vi "DAQ - Append NEW Data.vi"(0 "reference in":refnum<class "GSwFormDSP.lvclass">, 5 "error in (no error)":errorcluster, 7 "New Data":waveform(dbl)[](array[waveform])) -> (11 "Last Values":string[](array[string]), 13 "Time Offset":dbl, 14 "reference out":refnum<class "GSwFormDSP.lvclass">, 16 "Save to File":bool, 19 "error out":errorcluster)   [LabVIEW 2020, in "GSwFormDSP.lvclass"]
uses:
  GSwFormDSP.lvclass
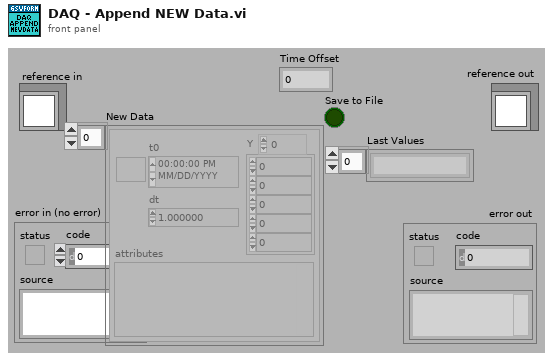
[diagram p1: front panel]
types:
  T1 = typedef "GSwFormDSP.lvclass/ObjectAttributes.ctl" = cluster{"Wform Ref":refnum<data-value>, "Nb Signals":i32, "Spectral Function Parameters":T2, "FFT":waveform(cdb)[], "Nb FFT":i32, "Nb Averages":i32[], "Reference Indexes":i32[], "Response Indexes":i32[], "Coherence":waveform(dbl)[], "TDF Parameters":T4, "DAQ":cluster{"Duration (sec)":dbl, "Buffer Size (Samples)":i32, "Offset (Samples)":i32}, "Filter Impulse Response (TDF)":waveform(dbl), "Sound Playback":T5}
  T2 = typedef "GSwFormDSP.lvclass/Spectral Parameters.ctl" = cluster{"Frequency resolution (Hz)":dbl, "Overlap":dbl, "Window":T3}
  T3 = typedef "NI_AALPro.lvlib/windowTd.ctl" = u32
  T4 = typedef "GSwFormDSP.lvclass/TDF Parameters.ctl" = cluster{"Filter":enum32{"Lowpass", "Highpass", "Bandpass", "Bandstop"}, "Type:":enum16{"Butterworth", "Chebyshev", "Inv Chebyshev", "Elliptic", "Bessel"}, "LP cutoff freq":dbl, "HP cutoff freq":dbl, "Order":i32, "passband ripple (dB)":dbl, "stopband attenuation (dB)":dbl, "Phaseless Filter":bool, "Include Fade IN and OUT":bool}
  T5 = typedef "GSwFormDSP.lvclass/Sound Playback.ctl" = cluster{"Timer start (ms)":u32, "task ID":T6, "Cursor Init Location (s)":dbl, "SC Volume":dbl}
  T6 = typedef "Sound Output Task ID.ctl" = u32
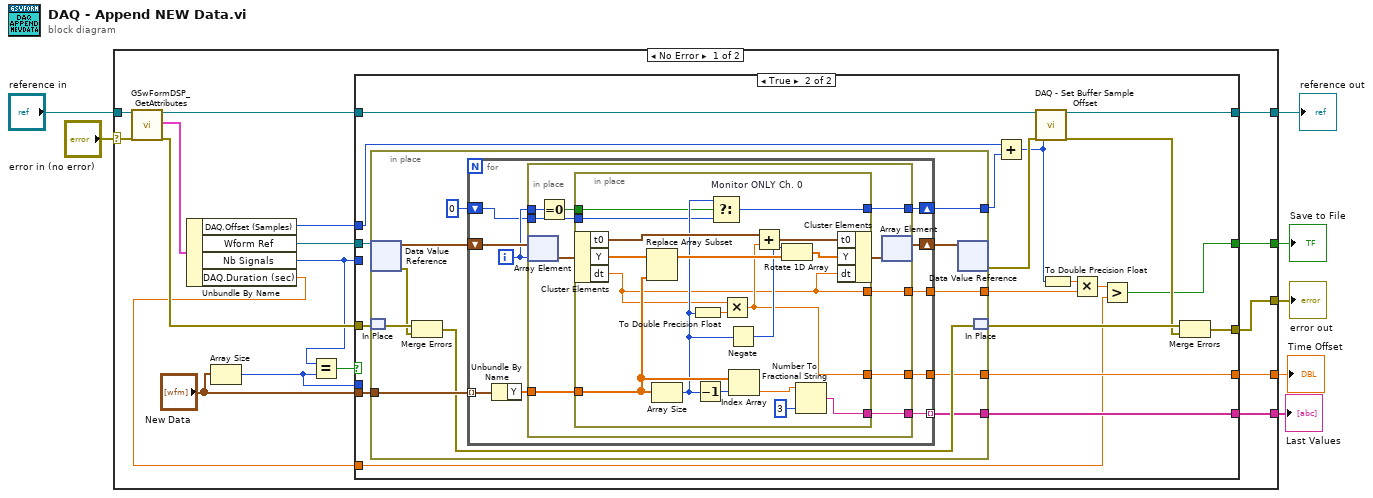
[diagram p0: block diagram]
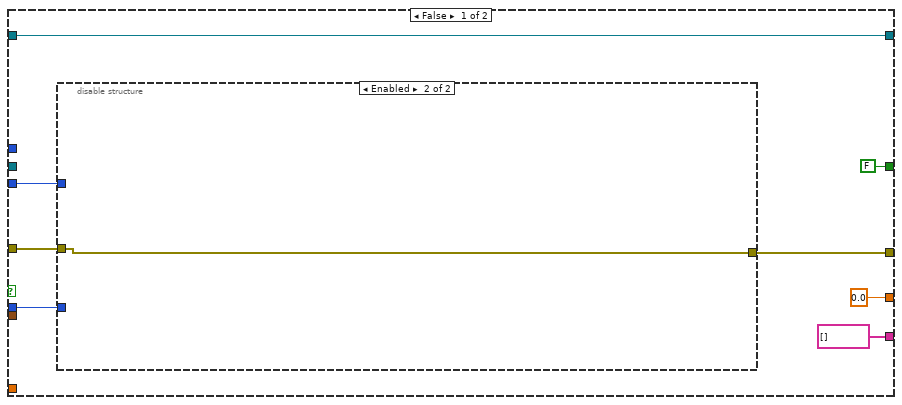
[diagram p2: hidden frame]
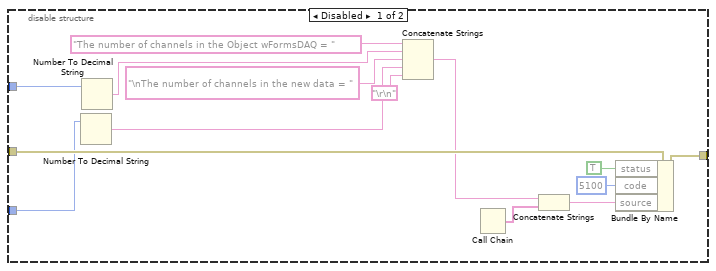
[diagram p3: hidden frame]
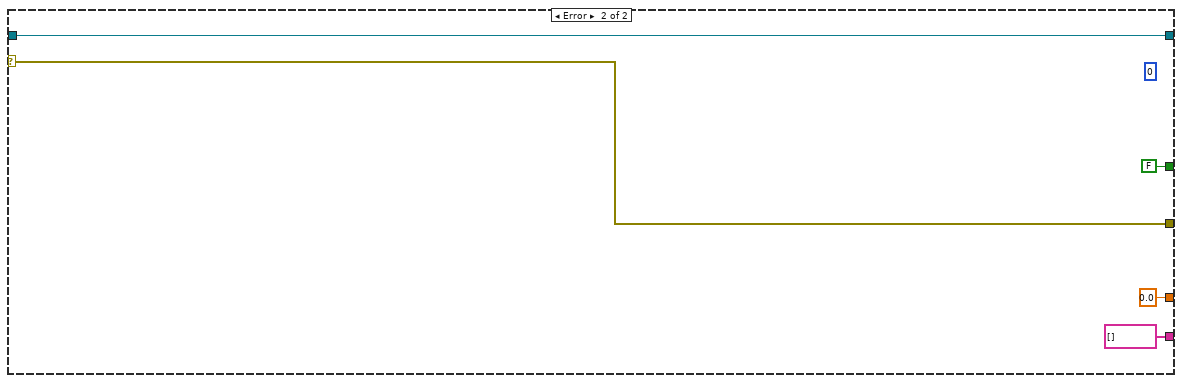
[diagram p4: hidden frame]
diagram:
  n1 = case shown="No Error" "error in (no error)" {
    selector: "error in (no error)" -> [w24 w120]
    tunnel: [w15 w120] -> w6
    tunnel: [w12 w119] -> w4
    tunnel: "reference in" -> [w23 w119]
    tunnel: [w14 0.0] -> w3
    tunnel: [w13 string[] []] -> w2
    tunnel: [w10 FALSE] -> w1
    frame No Error {
      n2 = call "GSwFormDSP_GetAttributes.vi"("reference in"=w23, "error in (no error)"=w24) -> ("reference out"=w21:refnum<class "GSwFormDSP.lvclass">, "attributes"=w22:T1, "error out"=w20:errorcluster)  [unwired: 14 in, 1 out]
      n3 = Unbundle By Name(w22) -> ("DAQ.Offset (Samples)"=w16:i32, "Wform Ref"=w17:refnum<data-value>, "Nb Signals"=w9:i32, "DAQ.Duration (sec)"=w11:dbl)
      n4 = Array Size(array="New Data") -> (size(s)=w8:i32)
      n5 = Equal?(x=w9, y=w8) -> (x = y?=w18:bool)
      n6 = case shown="True" w18 {
        tunnel: w17 -> [_ w66]
        tunnel: w20 -> [w32 w65]
        tunnel: [w31 w63] -> w15
        tunnel: "New Data" -> [_ w62]
        tunnel: [0.0 w61] -> w14
        tunnel: [string[] [] w60] -> w13
        tunnel: w16 -> [_ w55]
        tunnel: w21 -> [w28 w59]
        tunnel: [w28 w56] -> w12
        tunnel: w11 -> [_ w49]
        tunnel: [FALSE w48] -> w10
        tunnel: w9 -> [w26 _]
        tunnel: w8 -> [w25 _]
        frame False {
          n7 = disable-structure shown="Enabled" {
            disable-tunnel: w32 -> [w46 w47]
            disable-tunnel: [w44 w47] -> w31
            disable-tunnel: w26 -> [w40 _]
            disable-tunnel: w25 -> [w37 _]
            frame Disabled {
              n8 = Number To Decimal String(number=w37) -> (decimal integer string=w36:string)  [unwired: 1 in]
              n9 = Number To Decimal String(number=w40) -> (decimal integer string=w38:string)  [unwired: 1 in]
              n10 = Concatenate Strings("The number of channels in the Object wFormsDAQ = " ("source"), w38, "\nThe number of channels in the new data = " ("source"), w36, "\r\n") -> (w33:string)
              n11 = Call Chain() -> (call chain=w42:string[])
              n12 = Concatenate Strings(w33, w42) -> (w41:string)
              n13 = Bundle By Name(cluster=w46, "status"=TRUE, "code"=5100, "source"=w41) -> (w44:errorcluster)
            }
            frame Enabled {
            }
          }
        }
        frame True {
          n14 = in-place {
            in-place-border: w62 -> [w73]
            in-place-border: [w71] -> w61
            in-place-border: [w70] -> w60
            in-place-border: [w69] -> w54
            in-place-border: [w67] -> w51
            n15 = in-place-dvr #1(w66) -> (w75:waveform(dbl)[], w76:errorcluster)
            n16 = in-place-match #2(w65) -> (w77:errorcluster)
            n17 = Merge Errors(w77, w76) -> (w72:errorcluster)
            n18 = for {
              shift-right: [w86] -> w74
              shift-left: w75 -> [w87]
              tunnel: w73 -> [w85] mode=indexing
              tunnel: [w83] -> w71
              tunnel: [w82] -> w70 mode=indexing
              shift-right: [w81] -> w69
              shift-left: 0 -> [w79]
              tunnel: [w78] -> w67
              i -> [w80]
              n19 = Unbundle By Name(w85) -> ("Y"=w84:dbl[])
              n20 = in-place {
                in-place-border: w84 -> [w96]
                in-place-border: [w94] -> w83
                in-place-border: [w93] -> w82
                in-place-border: [w92] -> w81
                in-place-border: w80 -> [w91]
                in-place-border: w79 -> [w89]
                in-place-border: [w88] -> w78
                n21 = in-place-array #3(w87, w80) -> (w97:waveform(dbl))
                n22 = Equal To 0?(x=w91) -> (x = 0?=w90:bool)
                n23 = in-place {
                  in-place-border: w96 -> [w108]
                  in-place-border: [w109] -> w94
                  in-place-border: [w104] -> w93
                  in-place-border: [w100] -> w92
                  in-place-border: w90 -> [w101]
                  in-place-border: w89 -> [w99]
                  in-place-border: [w98] -> w88
                  n24 = in-place-cluster #4(w97) -> ("t0"=w111:timestamp, "Y"=w115:dbl[], "dt"=w98:dbl)
                  n25 = Replace Array Subset(array=w115, new element=w108) -> (w114:dbl[])  [unwired: 1 in]
                  n26 = Array Size(array=w108) -> (size(s)=w102:i32)
                  n27 = To Double Precision Float(number=w102) -> (double precision float=w112:dbl)
                  n28 = Decrement(x=w102) -> (x-1=w107:i32)
                  n29 = Select "Monitor ONLY Ch. 0"(t=w102, s=w101, f=w99) -> (s? t:f=w100:i32)
                  n30 = Multiply(x=w98, y=w112) -> (x*y=w109:dbl)
                  n31 = Negate(x=w102) -> (-x=w113:i32)
                  n32 = Index Array(array=w108, index=w107) -> (element=w106:dbl)
                  n33 = Add(x=w111, y=w109) -> (x+y=w110:timestamp)
                  n34 = Rotate 1D Array(1:w114, 2:w113) -> (0:w103:dbl[])
                  n35 = Number To Fractional String(number=w106, precision (6)=i16 3) -> (F-format string=w104:string)  [unwired: 2 in]
                  n36 = in-place-cluster #4("t0"=w110, "Y"=w103, "dt"=w98) -> (w95:waveform(dbl))
                }
                n37 = in-place-array #3(w95) -> (w86:waveform(dbl)[])  [unwired: 1 out]
              }
            }
            n38 = in-place-dvr #1(w74) -> (w58:errorcluster)  [unwired: 1 out]
            n39 = in-place-match #2(w72) -> (w64:errorcluster)
          }
          n40 = Add(x=w55, y=w54) -> (x+y=w53:i32)
          n41 = call "DAQ - Set Buffer Sample Offset.vi"("reference in"=w59, "error in (no error)"=w58, "DAQ.Offset (Samples)"=w53) -> ("reference out"=w56:refnum<class "GSwFormDSP.lvclass">, "error out"=w57:errorcluster)  [unwired: 15 in]
          n42 = To Double Precision Float(number=w53) -> (double precision float=w52:dbl)
          n43 = Multiply(x=w52, y=w51) -> (x*y=w50:dbl)
          n44 = Greater?(x=w50, y=w49) -> (0:w48:bool)
          n45 = Merge Errors(w64, w57) -> (w63:errorcluster)
        }
      }
    }
    frame Error {
      (unwired) 0
    }
  }
  "error out" <- w6
  "reference out" <- w4
  "Time Offset" <- w3
  "Last Values" <- w2
  "Save to File" <- w1
